vi "Occurence-Wait.vi"(2 "occurrence":refnum<k4>, 9 "error out":errorcluster caption="error in (no error)") -> (6 "error in (no error)":errorcluster caption="error out")   [LabVIEW 2009]
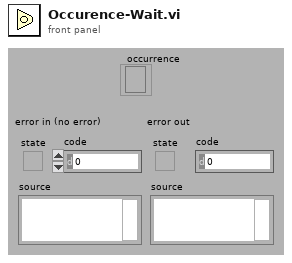
[diagram p1: front panel]
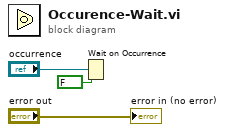
[diagram p0: block diagram]
diagram:
  n1 = Wait on Occurrence(1:FALSE ("ignorer précédent (V)"), 2:"occurrence") -> ()  [unwired: 2 out]
  "error in (no error)" <- "error out"
